vi "PolRead-C.vi"(0 "VISA resource name":refnum<visa-resource-name>, 1 "Byte Sum":i32, 2 "error in (no error)":errorcluster) -> (3 "VISA resource name out":refnum<visa-resource-name>, 4 "Polhemus Output":string, 5 "Time":u32, 6 "error out":errorcluster)   [LabVIEW 2012]
doc: "Waits for an incoming byte from the Polhemus then reads the specified number of bytes. Returns the output directly and the time (in arbitrary ms) when the first byte was received."
uses:
  <vilib>/Instr/_visa.llb/Select Event Type.ctl
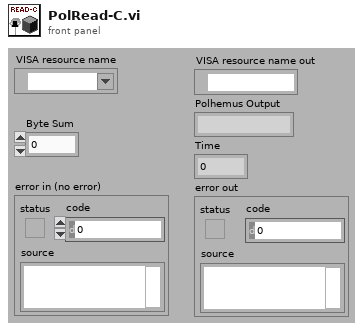
[diagram p1: front panel]
types:
  T1 = typedef "Select Event Type.ctl" = u32
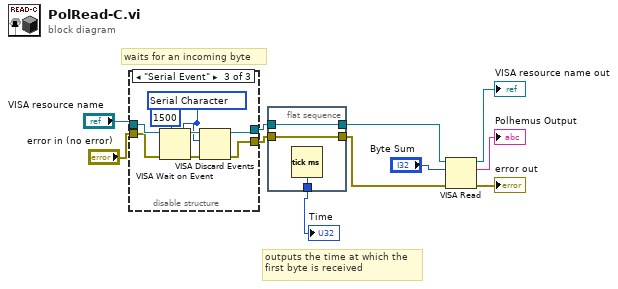
[diagram p0: block diagram]
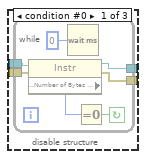
[diagram p2: hidden frame]
diagram:
  # "outputs the time at which the\nfirst byte is received"
  # "waits for an incoming byte"
  n1 = disable-structure shown="\"Serial Event\"" {
    disable-tunnel: "error in (no error)" -> [w15 w23 w31]
    disable-tunnel: "VISA resource name" -> [w14 w24 w32]
    disable-tunnel: [w13 w24 w27] -> w4
    disable-tunnel: [w12 w23 w28] -> w3
    frame condition #0 {
      n2 = while {
        tunnel: w15 -> [w20]
        tunnel: w14 -> [w19]
        tunnel: [w18] -> w13
        tunnel: [w17] -> w12
        stop <- w21 continue-if-true
        n3 = property class="Instr"(reference=w19, error in=w20) -> (reference out=w18:refnum<visa-resource-name>, error out=w17:errorcluster, "Serial Settings:Number of Bytes at Serial Port"=w22:u32)
        n4 = Wait (ms)(milliseconds to wait=u32 0) -> ()  [unwired: 1 out]
        n5 = Equal To 0?(x=w22) -> (x = 0?=w21:bool)
      }
    }
    frame condition #1 {
    }
    frame condition #2 (active) {
      w26 = T1 1073684533 items=["Service Request"=1073684491, "Trigger"=3221168138, "Clear"=1073684493, "VXI Signal"=1073684512, "VXI/VME Interrupt"=3221168161, "VXI/VME Sysfail"=1073684509, "VXI/VME Sysreset"=1073684510, "GPIB CIC"=1073684498, "GPIB Talk"=1073684499, "GPIB Listen"=1073684500, "PXI Interrupt"=1073684514, "Serial Break"=1073684515, "Serial TermChar"=1073684516, "Serial CTS"=1073684521, "Serial DSR"=1073684522, "Serial DCD"=1073684524, "Serial RI"=1073684526, "Serial Character"=1073684533, "USB Interrupt"=1073684535, "All Enabled"=1073709055] ("Event Type")
      n6 = VISA Wait on Event(7:u32 1500 ("timeout (0)"), 8:w31, 10:w26, 11:w32) -> (0:w29:errorcluster, 3:w30:refnum<visa-resource-name>)  [unwired: 1 in, 2 out]
      n7 = VISA Discard Events(8:w29, 10:w26, 11:w30) -> (0:w28:errorcluster, 3:w27:refnum<visa-resource-name>)  [unwired: 1 in]
    }
  }
  n8 = flat-sequence {
    tunnel: [w35] -> w8
    tunnel: [w34] -> w7
    tunnel: w4 -> [w34]
    tunnel: [w33] -> w6
    tunnel: w3 -> [w33]
    frame #0 {
      n9 = Tick Count (ms)() -> (millisecond timer value=w35:u32)
    }
  }
  n10 = VISA Read(VISA resource name=w7, byte count="Byte Sum", error in (no error)=w6) -> (VISA resource name out=→"VISA resource name out":refnum<visa-resource-name>, read buffer=→"Polhemus Output":string, error out=→"error out":errorcluster)  [unwired: 1 out]
  "Time" <- w8
